vi "Get Messenger.vi"(8 "error in (no error)":errorcluster, 10 "Messenger In":refnum<class "Messenger.lvclass">, 11 "Root Actor in":refnum<class "Root Actor.lvclass">) -> (0 "error out":errorcluster, 3 "Root Actor out":refnum<class "Root Actor.lvclass">)   [LabVIEW 2019, in "Root Actor.lvclass"]
uses:
  Root Actor.lvclass
  C:/Users/iio/Desktop/NTHU Brain Center/General Library/Ancestor Class/Actor/System Actor/System Actor.lvclass
  Messenger/Messenger/Messenger.lvclass
  Root Actor.lvclass/Root Actor.ctl
  System Actor/System Actor.lvclass/System Actor.ctl
  System Actor/Protected Data/Write Messenger Reference.vi
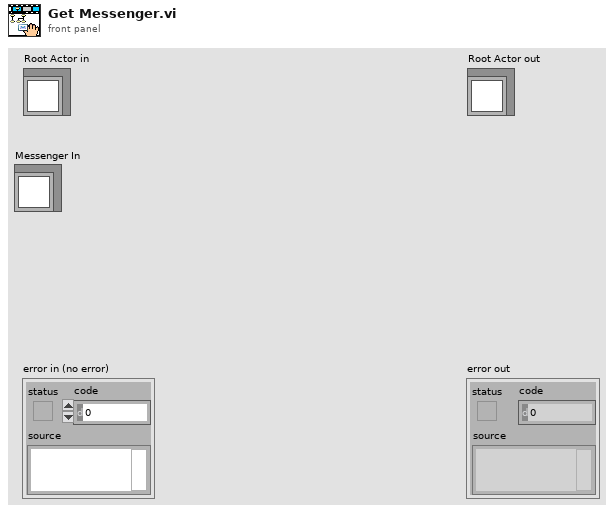
[diagram p1: front panel]
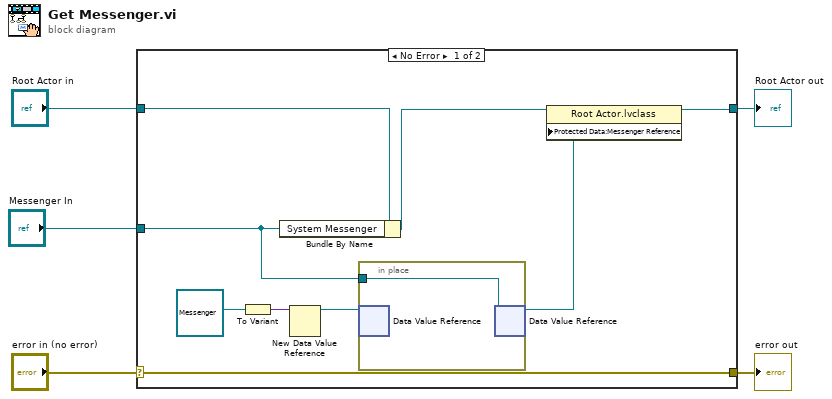
[diagram p0: block diagram]
diagram:
  n1 = case shown="No Error" "error in (no error)" {
    selector: "error in (no error)" -> [w14 w17]
    tunnel: [w14 w17] -> w4
    tunnel: [w11 w16] -> w2
    tunnel: "Root Actor in" -> [w13 w16]
    tunnel: "Messenger In" -> [w7 _]
    frame No Error {
      n2 = To Variant(anything=refnum<class "Messenger.lvclass"> refnum ("Messenger.lvclass")) -> (Variant=w10:variant)
      n3 = Bundle By Name(cluster=w13, "System Messenger"=w7) -> (w12:refnum<class "Root Actor.lvclass">)
      n4 = New Data Value Reference(data value=w10) -> (data value reference=w8:refnum<data-value>)  [unwired: 1 in, 1 out]
      n5 = in-place {
        in-place-border: w7 -> [w15]
        n6 = in-place-dvr #1(w8) -> ()  [unwired: 2 out]
        n7 = in-place-dvr #1(w15) -> (w6:refnum<data-value>)  [unwired: 1 out]
      }
      n8 = property class="Root Actor.lvclass"(reference=w12, "Protected Data:Messenger Reference"=w6) -> (reference out=w11:refnum<class "Root Actor.lvclass">)  [unwired: 1 in, 1 out]
    }
    frame Error {
    }
  }
  "error out" <- w4
  "Root Actor out" <- w2
